vi "putDynamicData.vi"(8 "error in (no error)":errorcluster, 10 "TelemetryDynamicData":T1, 11 "M1M3SAL in":refnum<class "M1M3SAL.lvclass">) -> (0 "error out":errorcluster, 3 "M1M3SAL out":refnum<class "M1M3SAL.lvclass">)   [LabVIEW 2016, in "M1M3SupportCommunicator.lvlib" / "M1M3SAL.lvclass"]
uses:
  M1M3SAL.lvclass
  DataTypes/Topics/TelemetryDynamicData.ctl
  DataTypes/Topics/Parts/Timestamp.ctl
  DataTypes/MessageHeader.ctl
  DataTypes/MessageTypes.ctl
  DataTypes/MessageTopics.ctl
  M1M3SAL.lvclass/M1M3SAL.ctl
  writeU8.vi
  writeI32.vi
  M1M3SupportCommunicator.lvlib
  DataTypes/Topics/M1M3SupportTopics.lvlib
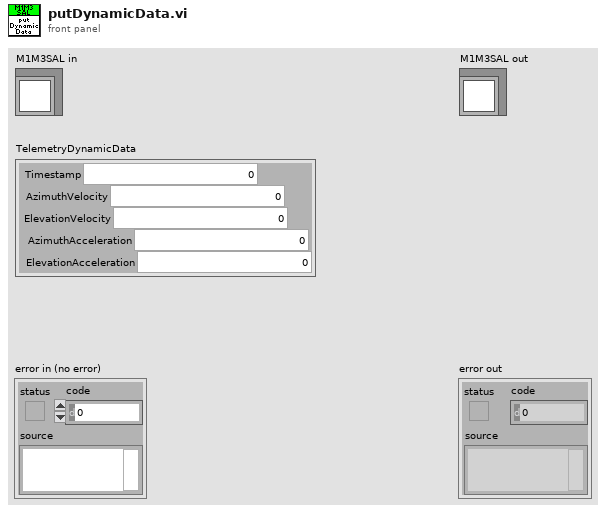
[diagram p1: front panel]
types:
  T1 = typedef "M1M3SupportTopics.lvlib/TelemetryDynamicData.ctl" = cluster{"Timestamp":T2, "AzimuthVelocity":dbl, "ElevationVelocity":dbl, "AzimuthAcceleration":dbl, "ElevationAcceleration":dbl}
  T2 = typedef "M1M3SupportTopics.lvlib/Timestamp.ctl" = dbl
  T3 = typedef "M1M3SupportCommunicator.lvlib/MessageHeader.ctl" = cluster{"Type":T4, "Topic":T5, "Size":i32}
  T4 = typedef "M1M3SupportCommunicator.lvlib/MessageTypes.ctl" = enum8{"None", "PutSample", "GetNextSample", "LogEvent", "GetEvent", "IssueCommand", "CommandId", "WaitForCompletion", "AcceptCommand", "AckCommand"}
  T5 = typedef "M1M3SupportCommunicator.lvlib/MessageTopics.ctl" = enum8{"None", "ForceActuatorData", "MirrorForceData", "HardpointData", "AirData", "DynamicData", "FPGAData", "IMSData", "ForceActuatorStatus", "ElevationData", "HardpointStatus", "HardpointActuatorChase", "AirStatus", "ForceActuatorSafetyChecks", "ForceActuatorTest", "ActuatorBroadcastCounter", "StatusChecks", "CellChecks", "HardpointActuatorBreakaway", "RaiseMirrorComplete", "ILCCommunication", "ElevationAngleChecks", "DetailedState", "ServoLoops", "ForceActuatorInfo", "LowerMirrorComplete", "HardpointActuatorInfo", "SettingsApplied", "ErrorCode", "StartupChecks", "SummaryState", "SettingVersions", "ActuatorTestStatus", "AppliedSettingsMatchStart", "Enable", "EnterMaintenance", "Standby", "AbortLowerM1M3", "ApplyAberrationByForces", "ApplyAOSCorrectionByBendingModes", "ClearAOSCorrection", "Start", "RaiseM1M3", "TestForceActuator", "LowerM1M3", "ApplyAOSCorrectionByForces", "Disable", "ApplyAberationByBendingMode", "TestHardpoint", "ManipulateM1M3", "ClearAberration", "Exit", "TestAir", "AbortRaiseM1M3", "MoveHardpointActuators", "ExitMaintenance", "Shutdown"}
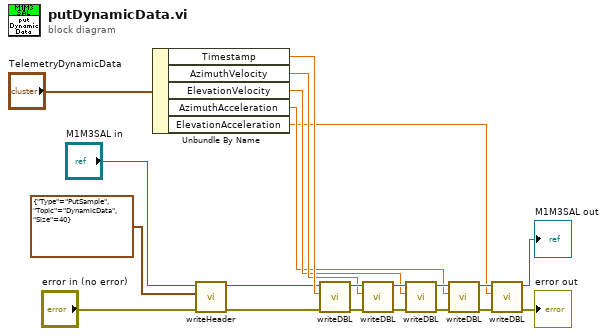
[diagram p0: block diagram]
diagram:
  n1 = Unbundle By Name("TelemetryDynamicData") -> ("Timestamp"=w10:T2, "AzimuthVelocity"=w9:dbl, "ElevationVelocity"=w8:dbl, "AzimuthAcceleration"=w7:dbl, "ElevationAcceleration"=w6:dbl)
  n2 = call "writeHeader.vi"("error in (no error)"="error in (no error)", "MessageHeader"=T3 {"Type"=enum."PutSample", "Topic"=enum."DynamicData", "Size"=40}, "M1M3SAL in"="M1M3SAL in") -> ("error out"=w3:errorcluster, "M1M3SAL out"=w5:refnum<class "M1M3SAL.lvclass">)  [unwired: 7 in]
  n3 = call "writeDBL.vi"("error in (no error)"=w3, "Input"=w10, "M1M3SAL in"=w5) -> ("error out"=w18:errorcluster, "M1M3SAL out"=w17:refnum<class "M1M3SAL.lvclass">)  [unwired: 7 in]
  n4 = call "writeDBL.vi"("error in (no error)"=w18, "Input"=w9, "M1M3SAL in"=w17) -> ("error out"=w11:errorcluster, "M1M3SAL out"=w12:refnum<class "M1M3SAL.lvclass">)  [unwired: 7 in]
  n5 = call "writeDBL.vi"("error in (no error)"=w11, "Input"=w8, "M1M3SAL in"=w12) -> ("error out"=w16:errorcluster, "M1M3SAL out"=w15:refnum<class "M1M3SAL.lvclass">)  [unwired: 7 in]
  n6 = call "writeDBL.vi"("error in (no error)"=w16, "Input"=w7, "M1M3SAL in"=w15) -> ("error out"=w14:errorcluster, "M1M3SAL out"=w13:refnum<class "M1M3SAL.lvclass">)  [unwired: 7 in]
  n7 = call "writeDBL.vi"("error in (no error)"=w14, "Input"=w6, "M1M3SAL in"=w13) -> ("error out"=→"error out":errorcluster, "M1M3SAL out"=→"M1M3SAL out":refnum<class "M1M3SAL.lvclass">)  [unwired: 7 in]
